vi "WPI_DigitalModuleSetDIO.vi"(8 "error in (no error)":errorcluster, 9 "Value":bool, 10 "DIOChannel":T1=enum."DIO 1", 11 "DigitalModuleDevRef":T2) -> (0 "error out":errorcluster, 3 "DigitalModuleDevRef":T2)   [LabVIEW 2017]
doc: "This software is licensed. Open the labview\\readme\\WPI Robotics Library Open Source License.txt file for more information."
uses:
  <vilib>/Rock Robotics/WPI/DigitalModule/WPI_DigitalModuleDeviceRef.ctl
  <vilib>/Rock Robotics/SystemInterfaces/DIO/FPGA_DIOChannel.ctl
  <vilib>/Rock Robotics/SystemInterfaces/System/FPGA_SystemGet.vi
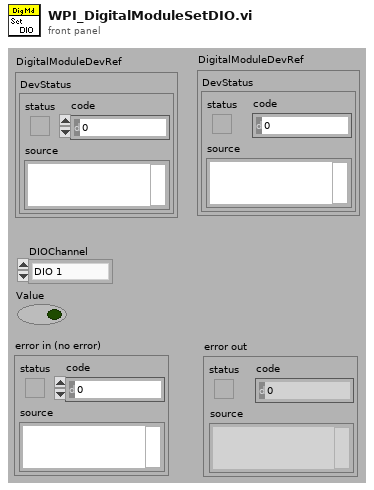
[diagram p1: front panel]
types:
  T1 = typedef "FPGA_DIOChannel.ctl" = enum8{"DIO 0", "DIO 1", "DIO 2", "DIO 3", "DIO 4", "DIO 5", "DIO 6", "DIO 7", "DIO 8", "DIO 9", "DIO MXP 0", "DIO MXP 1", "DIO MXP 2", "DIO MXP 3", "DIO MXP 4", "DIO MXP 5", "DIO MXP 6", "DIO MXP 7", "DIO MXP 8", "DIO MXP 9", "DIO MXP 10", "DIO MXP 11", "DIO MXP 12", "DIO MXP 13", "DIO MXP 14", "DIO MXP 15", "SPI Port CS1", "SPI Port CS2", "SPI Port CS3", "SPI Port MISO", "SPI Port MOSI", "Invalid"}
  T2 = typedef "WPI_DigitalModuleDeviceRef.ctl" = cluster{"DevStatus":errorcluster}
  T3 = typedef "FPGA_DIODevRef.ctl" = cluster{"DevStatus":errorcluster}
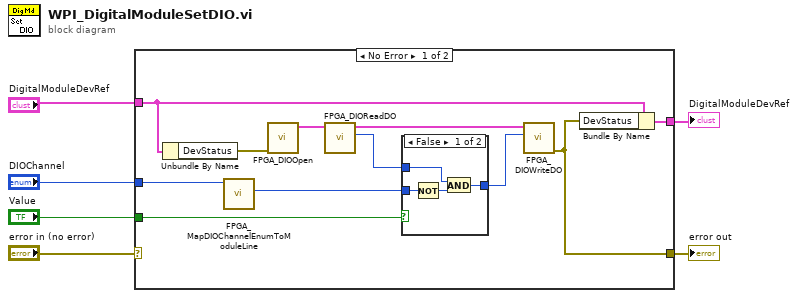
[diagram p0: block diagram]
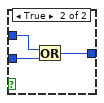
[diagram p2: hidden frame]
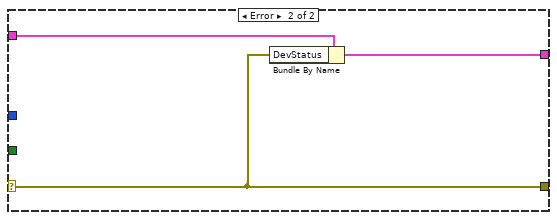
[diagram p3: hidden frame]
diagram:
  n1 = case shown="No Error" "error in (no error)" {
    selector: "error in (no error)" -> [_ w25]
    tunnel: "DigitalModuleDevRef" -> [w17 w27]
    tunnel: [w16 w26] -> w2
    tunnel: [w12 w25] -> w5
    tunnel: "Value" -> [w15 _]
    tunnel: "DIOChannel" -> [w11 _]
    frame No Error {
      n2 = Unbundle By Name(w17) -> ("DevStatus"=w13:errorcluster)
      n3 = call <vilib>:"FPGA_MapDIOChannelEnumToModuleLine.vi"("DIOChannel"=w11) -> ("ActualDIOBitMask(U32)"=w10:u32)  [unwired: 10 out]
      n4 = call <vilib>:"FPGA_DIOOpen.vi"("error in (no error)"=w13) -> ("DIODeviceRef"=w9:T3)  [unwired: 1 in, 9 out]
      n5 = call <vilib>:"FPGA_DIOReadDO.vi"("DIODeviceRef In"=w9) -> ("DO"=w7:u32, "DIODeviceRef Out"=w8:T3)  [unwired: 1 in, 8 out]
      n6 = case shown="False" w15 {
        tunnel: w7 -> [w19 w23]
        tunnel: w10 -> [w21 w24]
        tunnel: [w18 w22] -> w14
        frame False {
          n7 = Not(x=w21) -> (.not. x?=w20:u32)
          n8 = And(x=w19, y=w20) -> (x .and. y?=w18:u32)
        }
        frame True {
          n9 = Or(x=w23, y=w24) -> (x .or. y?=w22:u32)
        }
      }
      n10 = call <vilib>:"FPGA_DIOWriteDO.vi"("DO"=w14, "DIODeviceRef"=w8) -> ("error out"=w12:errorcluster)  [unwired: 1 in, 8 out]
      n11 = Bundle By Name(cluster=w17, "DevStatus"=w12) -> (w16:T2)
    }
    frame Error {
      n12 = Bundle By Name(cluster=w27, "DevStatus"=w25) -> (w26:T2)
    }
  }
  "error out" <- w5
  "DigitalModuleDevRef" <- w2
